vi "Main_Framework.vi"() -> (0 "error out":errorcluster, 3 "output anno":T1(plugin-control))   [LabVIEW 2021, in "Framework_lib.lvlib"]
doc: "This example demonstrates how to call a Python function and pass arguments as numpy arrays. It uses a python function to compute the product of two matrices."
uses:
  QMH/Framework_lib.lvlib
  QMH/QMH_Producer_type.ctl
  FW_Image_resultant_data.ctl
  <vilib>/vision/Image Controls.llb/IMAQ Image.ctl
  QMH/QMH_references_enum.ctl
  FW_Consumer_Data.ctl
  FW_pyAnnotation_parameters.ctl
  FW_producer_Cluster.ctl
  FW_producer_Data.ctl
  FW_Results_Data.ctl
  FW_Frames_Data.ctl
  QMH_producer_enum.ctl
  64de032f-f1bc-4223-962d-436fd60f823b.vi
  a236fdb2-980f-4409-8fc5-f52671132e3e.vi
panel:
  in  "Tab Control":enum32{"Original", "BirdEye", "Final"}(tab)
  out "Input Annotation":T1(plugin-control)
  out "Input SUT":T1(plugin-control)
  out "output SUT":T1(plugin-control)
  out "final 2":T1(plugin-control)
  out "final":T1(plugin-control)
  out "Paused_ann":bool
  out "Paused":bool
  in  "Pause?":bool
  in  "PNG/AVI (F:JPG)":bool
  out "data":T5
  out "Message 2":string
  out "Message":string
  in  "Resume":bool
  out "Waveform Graph":sgl[][](graph)
  in  "Start":bool
  in  "Stop":bool
  out "elapsed_img2arr (ms) 2":u32
  out "elapsed_py (ms) 2":u32
  out "elapsed_py (ms)":u32
  out "elapsed_img2arr (ms)":u32
  in  "name or relative path":path[](array[path])=[path "D:/PELUSO/ITSligo/lectures_MENG/5-Thesis/project/test_hough"]
  out "elapsed_redraw":u32
  # "Main"
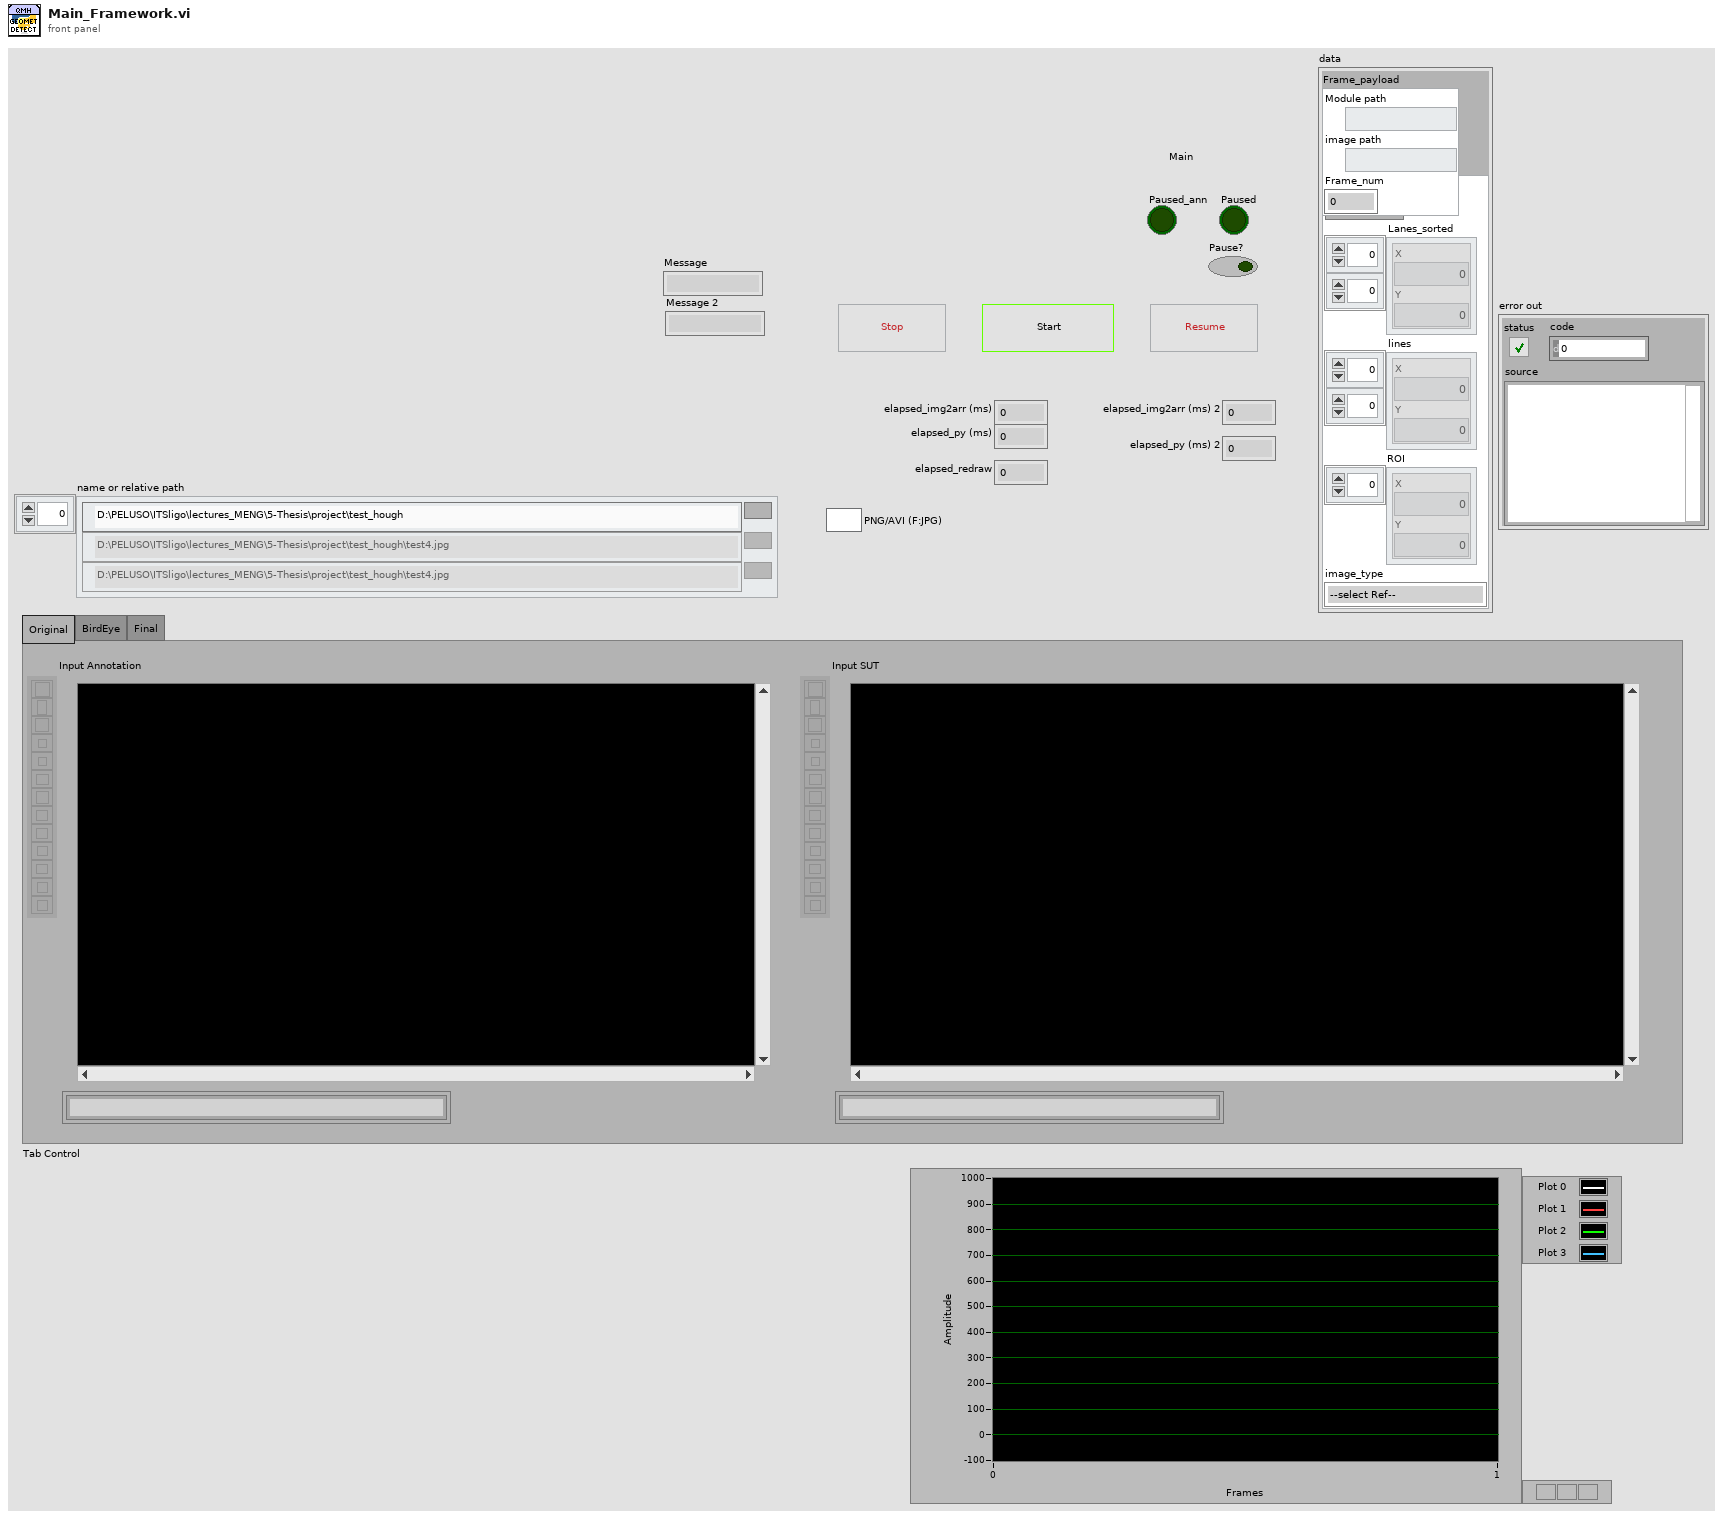
[diagram p1: front panel]
types:
  T1 = typedef "IMAQ Image.ctl" = refnum<image>
  T2 = typedef "Framework_lib.lvlib/QMH_Producer_type.ctl" = cluster{"Module path":path, "image path":path, "Frame_num":u16}
  T3 = typedef "Framework_lib.lvlib/FW_Image_resultant_data.ctl" = cluster{"Image_ref":T1, "Lanes_sorted":cluster{"X":dbl, "Y":dbl}[][], "lines":cluster{"X":dbl, "Y":dbl}[][], "ROI":cluster{"X":dbl, "Y":dbl}[], "image_type":T4}
  T4 = typedef "Framework_lib.lvlib/QMH_references_enum.ctl" = enum16{"--select Ref--", "Consumer_SUT", "Consumer_Annot", "Compute_Results"}
  T5 = cluster{"Frame_payload":T2, "image_resultant":T3}
  T6 = typedef "Framework_lib.lvlib/FW_Consumer_Data.ctl" = cluster{"Py session":refnum<k35>, "Image_orignal":T1, "Image_trans":T1, "ROI_params":T7, "Frame_payload":T2, "image_resultant":T3, "Paused":bool}
  T7 = typedef "Framework_lib.lvlib/FW_pyAnnotation_parameters.ctl" = cluster{"scale_w":dbl, "scale_h":dbl, "offset_X":dbl, "offset_Y":dbl, "Rho":dbl, "Theta":dbl, "Threshold":i32, "min_line_len":i32, "max_line_gap":i32}
  T8 = typedef "Framework_lib.lvlib/FW_Results_Data.ctl" = cluster{"Py session":refnum<k35>, "BirdEyeView_params":cluster{"P1":cluster{"x":i16, "y":i16}, "P2":cluster{"x":i16, "y":i16}, "Alfa":dbl}, "frames_Result":T9[]}
  T9 = typedef "Framework_lib.lvlib/FW_Frames_Data.ctl" = cluster{"Frame_payload":T2, "image_resultant":T3, "Image_Warp_perspective":T1, "Image_Warpped_BW":T1, "Warpped_detected_points":cluster{"X":sgl, "Y":sgl}[][]}
  T10 = cluster{"Global Rectangle":i32[], "Contours":cluster{"Contour Type":u32, "ROI Type":u32, "Points":i32[]}[]}
  T11 = cluster{"scale_w":dbl, "scale_h":dbl, "offset_X":dbl, "offset_Y":dbl, "min_line_len":dbl, "max_line_gap":dbl}
  T12 = typedef "Framework_lib.lvlib/FW_producer_Cluster.ctl" = cluster{"Py session":refnum<k35>, "start_time":u32, "process_running":T13[], "output cluster":T2}
  T13 = typedef "Framework_lib.lvlib/FW_producer_Data.ctl" = cluster{"Queue_Ref":T4, "running":bool}
  T14 = cluster{"Left Lane":cluster{"X":i32, "Y":i32}[], "Right Lane":cluster{"X":i32, "Y":i32}[]}
  T15 = cluster{"Module Path":path, "python_img_array":u8[][][], "Parameters in":variant}
  T16 = typedef "Framework_lib.lvlib/QMH_producer_enum.ctl" = enum16{"Idle", "Initialize", "Shutdown", "ERROR", "Stop", "Start", "Enqueue_frames", "Paused", "Resume"}
  T17 = cluster{"P1":cluster{"x":i16, "y":i16}, "P2":cluster{"x":i16, "y":i16}, "Alfa":dbl}
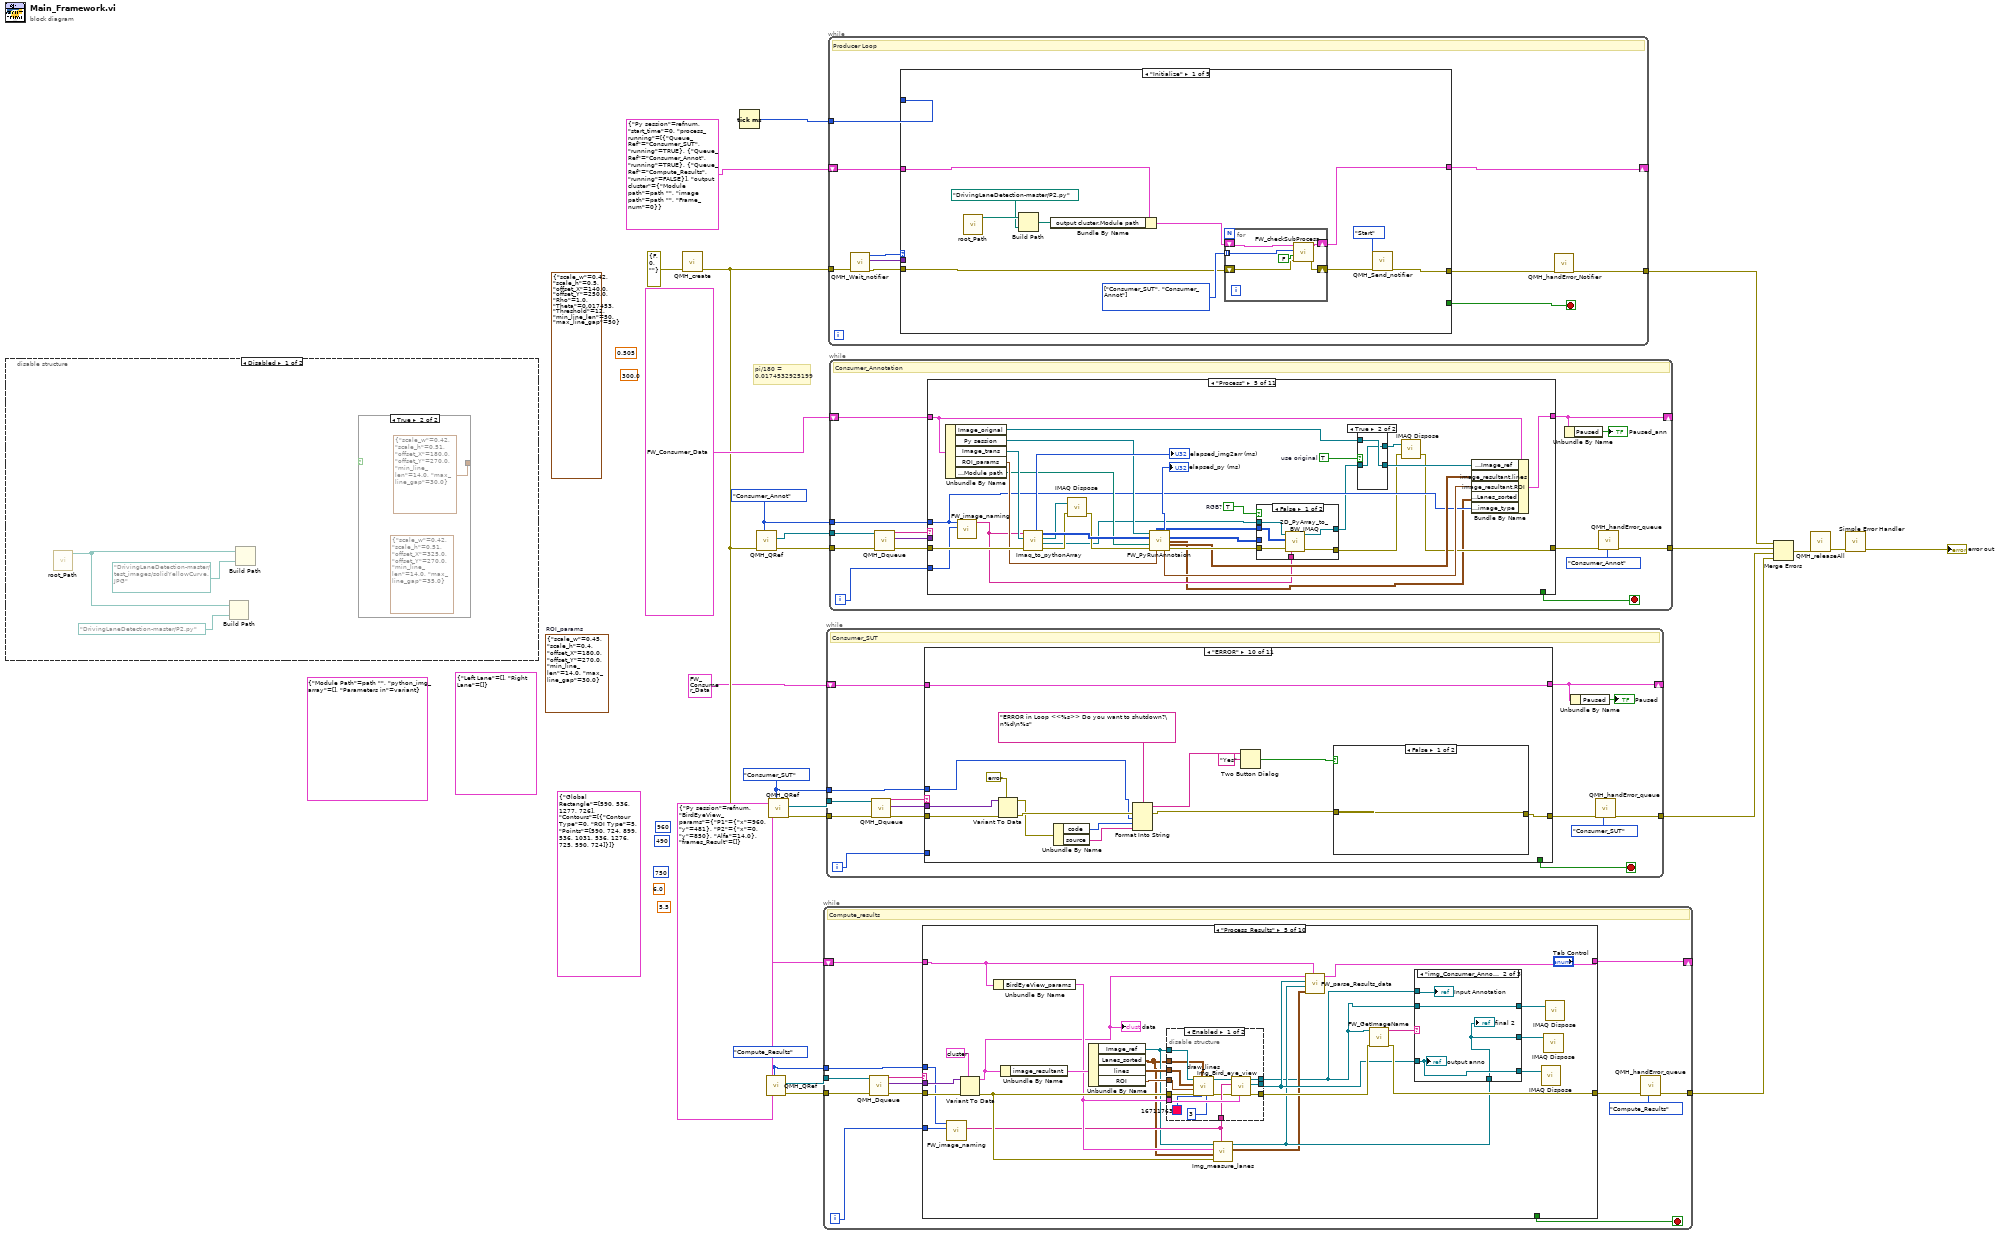
[diagram p0: block diagram]
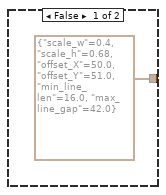
[diagram p2: hidden frame]
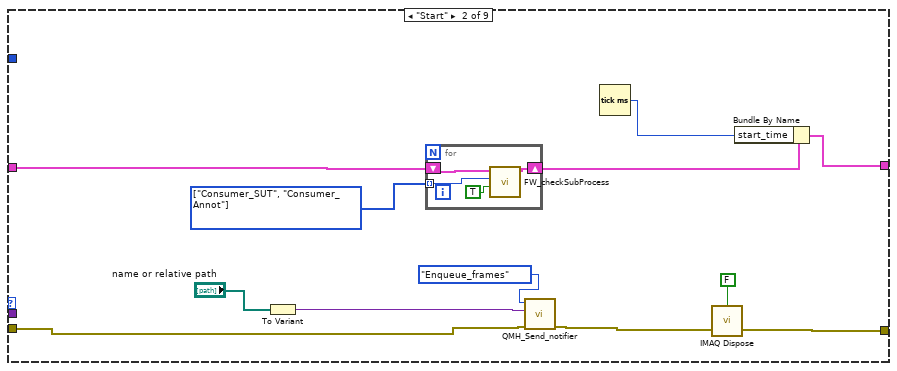
[diagram p4: hidden frame]
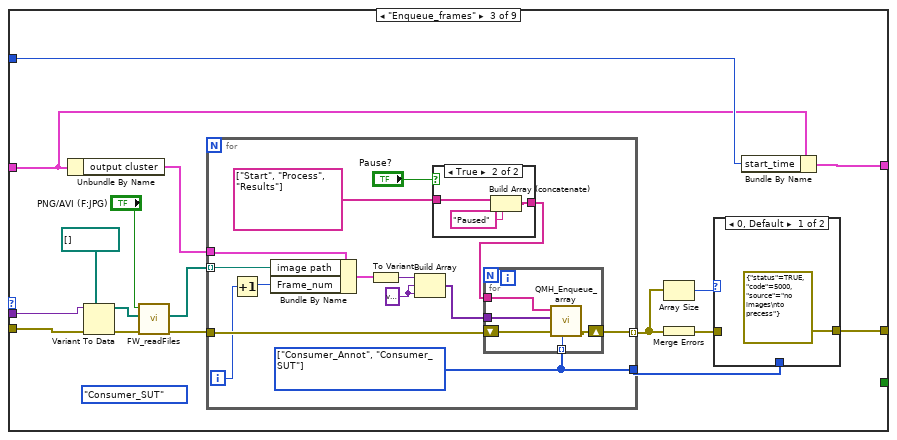
[diagram p5: hidden frame]
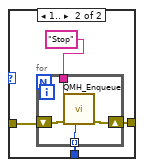
[diagram p6: hidden frame]
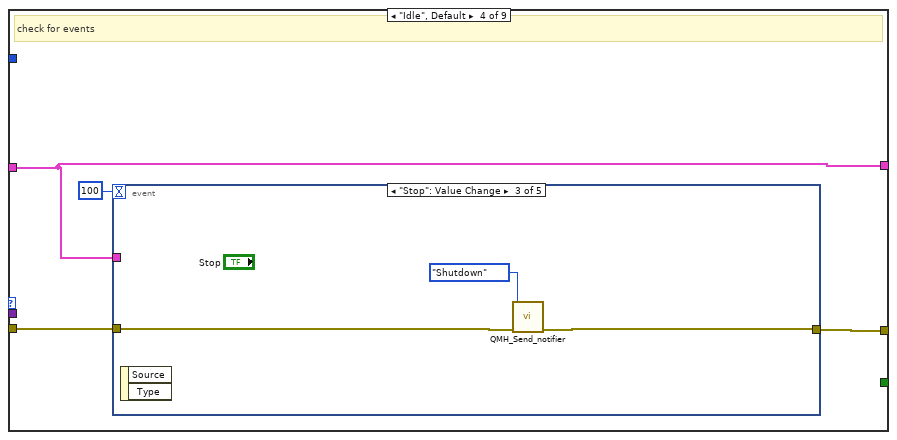
[diagram p8: hidden frame]
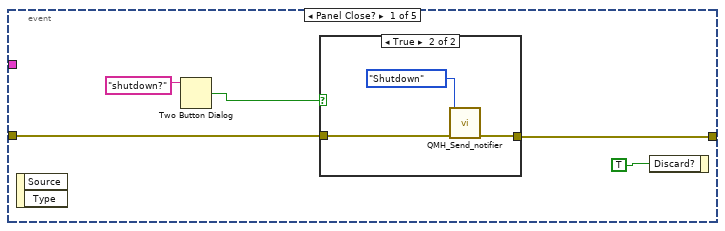
[diagram p9: hidden frame]
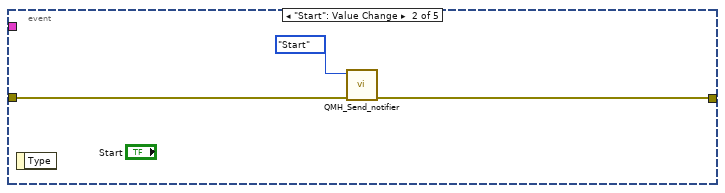
[diagram p11: hidden frame]
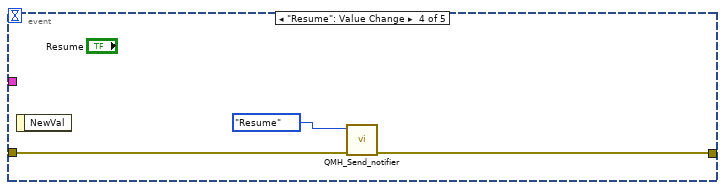
[diagram p12: hidden frame]
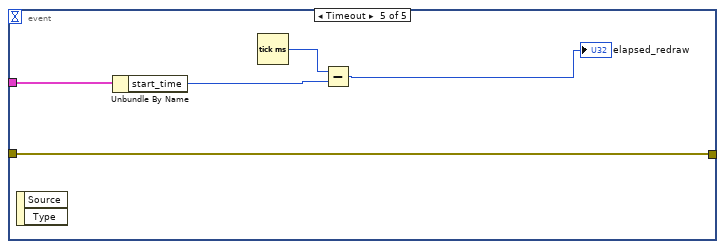
[diagram p13: hidden frame]
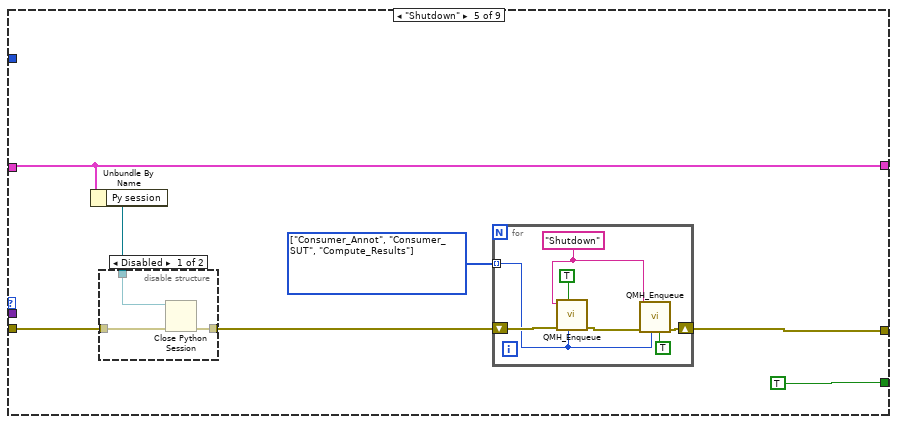
[diagram p14: hidden frame]
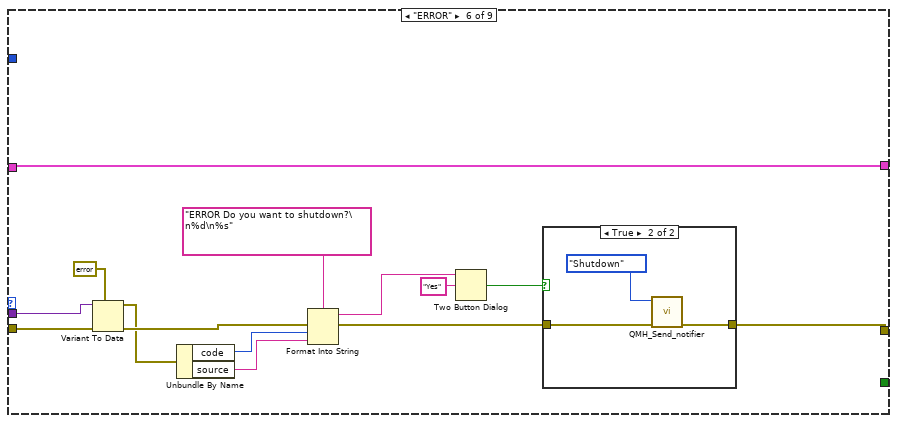
[diagram p16: hidden frame]
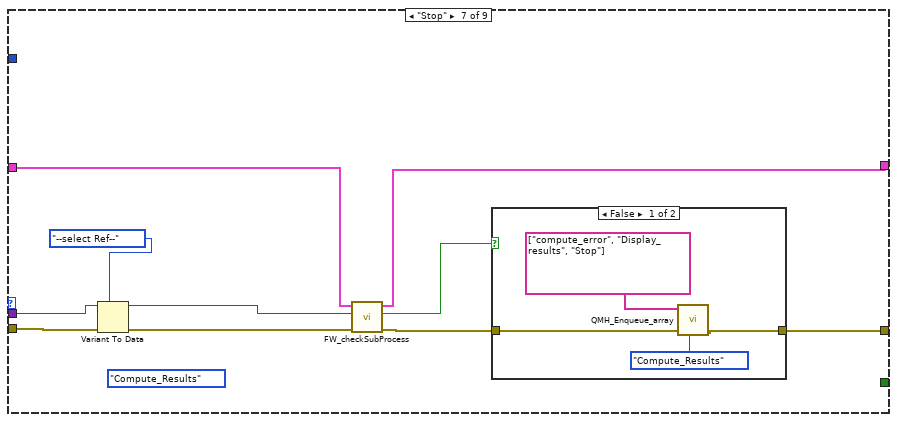
[diagram p18: hidden frame]
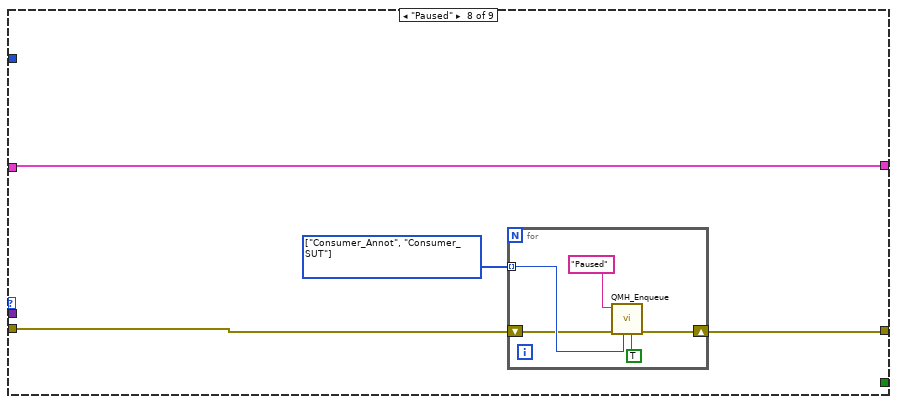
[diagram p20: hidden frame]
diagram:
  (unwired) 0.505 ("scale_h")
  (unwired) 5.5 ("Alfa")
  (unwired) i16 960 ("x")
  (unwired) i16 490 ("y")
  (unwired) 6.0 ("Alfa")
  (unwired) i16 750 ("y")
  (unwired) 300.0 ("offset_Y")
  (unwired) T7 {"scale_w"=0.42, "scale_h"=0.5, "offset_X"=140.0, "offset_Y"=250.0, "Rho"=1.0, "Theta"=0.017453, "Threshold"=12, "min_line_len"=50, "max_line_gap"=50} ("ROI_params")
  w5 = QMH_references_enum."Compute_Results" ("Enum")
  (unwired) T10 {"Global Rectangle"=[590, 536, 1277, 726], "Contours"=[{"Contour Type"=0, "ROI Type"=5, "Points"=[590, 724, 899, 536, 1031, 536, 1276, 725, 590, 724]}]} ("ROI")
  w9 = QMH_references_enum."Consumer_SUT" ("Enum")
  w10 = QMH_references_enum."Consumer_Annot" ("Enum")
  (unwired) T11 {"scale_w"=0.45, "scale_h"=0.4, "offset_X"=180.0, "offset_Y"=270.0, "min_line_len"=14.0, "max_line_gap"=30.0}  # ROI_params
  (unwired) T14 {"Left Lane"=[], "Right Lane"=[]}
  (unwired) T15 {"Module Path"=path "", "python_img_array"=[], "Parameters in"=variant}
  # "pi/180 =\n0.0174532925199"
  n1 = disable-structure shown="Disabled" {
    frame Disabled {
      n2 = call "root_Path.vi"() -> ("name or relative path"=w24:path)  [unwired: 11 in]
      n3 = Build Path(base path=w24, name or relative path=path "DrivingLaneDetection-master/P2.py") -> ()  [unwired: 1 out]
      n4 = Build Path(base path=w24, name or relative path=path "DrivingLaneDetection-master/test_images/solidYellowCurve.JPG") -> ()  [unwired: 1 out]
      n5 = case shown="True" {
        selector: _ -> [_ _]
        tunnel: [T11 {"scale_w"=0.4, "scale_h"=0.68, "offset_X"=50.0, "offset_Y"=51.0, "min_line_len"=16.0, "max_line_gap"=42.0} T11 {"scale_w"=0.42, "scale_h"=0.51, "offset_X"=180.0, "offset_Y"=270.0, "min_line_len"=14.0, "max_line_gap"=30.0}] -> _
        frame False {
        }
        frame True {
          (unwired) T11 {"scale_w"=0.42, "scale_h"=0.51, "offset_X"=325.0, "offset_Y"=270.0, "min_line_len"=14.0, "max_line_gap"=35.0}
        }
      }
    }
    frame Enabled {
    }
  }
  n6 = call "QMH_create.vi"("error in (no error)"=errorcluster {"status"=FALSE, "code"=0, "source"=""}) -> ("error out"=w4:errorcluster)  [unwired: 10 in]
  n7 = Tick Count (ms)() -> (millisecond timer value=w2:u32)
  n8 = call "QMH_QRef.vi"("Enum"=w10, "error in (no error)"=w4) -> ("error out"=w14:errorcluster, "Queue_ref"=w13:refnum<queue>)  [unwired: 7 in, 1 out]
  n9 = call "QMH_QRef.vi"("Enum"=w5, "error in (no error)"=w4) -> ("error out"=w7:errorcluster, "Queue_ref"=w6:refnum<queue>)  [unwired: 7 in, 1 out]
  n10 = call "QMH_QRef.vi"("Enum"=w9, "error in (no error)"=w4) -> ("error out"=w12:errorcluster, "Queue_ref"=w11:refnum<queue>)  [unwired: 7 in, 1 out]
  n11 = while {
    tunnel: w7 -> [w41]
    tunnel: [w33] -> w3
    shift-right: [w36] -> _
    shift-left: T8 {"Py session"=refnum, "BirdEyeView_params"={"P1"={"x"=960, "y"=481}, "P2"={"x"=0, "y"=850}, "Alfa"=14.0}, "frames_Result"=[]} -> [w37]
    tunnel: w6 -> [w31]
    tunnel: w5 -> [w30]
    i -> [w29]
    stop <- w35 stop-if-true
    # "Compute_results"
    n12 = call "QMH_Dqueue.vi"("error in (no error)"=w41, "Queue_ref"=w31) -> ("error out"=w40:errorcluster, "Payload"=w38:variant, "Message"=w39:string)  [unwired: 7 in]
    n13 = case shown="\"Process_Results\"" w39 {
      selector: w39 -> [w42 _ _ _ _ _ _ _ _ _]
      tunnel: w40 -> [w46 w49 w55 w69 w97 w126 w129 w136 w150 w170]
      tunnel: w38 -> [_ _ _ w67 w96 _ _ _ w149 _]
      tunnel: [w45 w49 w53 w70 w88 w126 w129 w135 w152 w169] -> w34
      tunnel: w37 -> [w48 w50 w54 w61 w83 w128 w130 w132 w161 w171]
      tunnel: [w48 w50 w52 w61 w82 w128 w130 w132 w161 w171] -> w36
      tunnel: [_ _ _ _ _ _ _ _ _ TRUE] -> w35
      tunnel: w30 -> [w43 _ _ w62 w91 _ _ w134 w148 _]
      tunnel: w29 -> [_ _ _ w63 w90 _ _ _ _ _]
      frame "", Default {
        n14 = Format Into String(format string="Loop <<%s>> : \nbad message: %s", error in=w46, w43, w42) -> (resulting string=w44:string, error out=w45:errorcluster)  [unwired: 1 in]
        n15 = One Button Dialog(message=w44) -> ()  [unwired: 1 in, 1 out]
      }
      frame "*IDLE*" {
        # "do nothing, just loop through"
      }
      frame "Initialize" {
        n16 = disable-structure shown="Disabled" {
          disable-tunnel: w55 -> [w58 w59]
          disable-tunnel: [w57 w59] -> w53
          disable-tunnel: [w56 _] -> w51
          frame Disabled {
            n17 = call "create python session.vi"("error in (no error)"=w58) -> ("error out"=w57:errorcluster, "session out"=w56:refnum<k35>)  [unwired: 8 in, 1 out]
          }
          frame Enabled {
          }
        }
        n18 = Bundle By Name(cluster=w54, "Py session"=w51) -> (w52:T8)
      }
      frame "Start" {
        w71 = "clear_buffer"  # function name
        n19 = Variant To Data(error in=w69, type=T2 {"Module path"=path "", "image path"=path "", "Frame_num"=0} ("output cluster"), Variant=w67) -> (data=w66:T2, error out=w68:errorcluster)
        n20 = call "FW_image_naming.vi"("Numeric"=w63, "Enum"=w62) -> ()  [unwired: 9 in, 1 out]
        n21 = Unbundle By Name(w61) -> ("Py session"=w60:refnum<k35>)
        n22 = Unbundle By Name(w66) -> ("Module path"=w65:path)  [unwired: 1 out]
        n23 = node(w60, w65, w71, w68) -> (w70:errorcluster)  [unwired: 2 in, 3 out]
      }
      frame "Process_Results" {
        n24 = call "FW_image_naming.vi"("Numeric"=w90, "Enum"=w91) -> ("String"=w84:string)  [unwired: 9 in]
        n25 = Variant To Data(error in=w97, type=T5 {"Frame_payload"={"Module path"=path "", "image path"=path "", "Frame_num"=0}, "image_resultant"={"Image_ref"=refnum, "Lanes_sorted"=[], "lines"=[], "ROI"=[], "image_type"=enum."--select Ref--"}} ("output cluster"), Variant=w96) -> (data=w77:T5, error out=w87:errorcluster)
        "data" <- w77
        n26 = Unbundle By Name(w83) -> ("BirdEyeView_params"=w85:T17)
        n27 = Unbundle By Name(w77) -> ("image_resultant"=w94:T3)
        n28 = Unbundle By Name(w94) -> ("Image_ref"=w81:T1, "Lanes_sorted"=w72:cluster{"X":dbl, "Y":dbl}[][], "lines"=w86:cluster{"X":dbl, "Y":dbl}[][], "ROI"=w93:cluster{"X":dbl, "Y":dbl}[])
        n29 = disable-structure shown="Enabled" {
          disable-tunnel: w93 -> [w111 _]
          disable-tunnel: [w110 w112] -> w89
          disable-tunnel: [w109 w113] -> w73
          disable-tunnel: w87 -> [w108 w112]
          disable-tunnel: w86 -> [w107 _]
          disable-tunnel: w85 -> [w106 _]
          disable-tunnel: w84 -> [w105 _]
          disable-tunnel: w81 -> [w104 w113]
          disable-tunnel: [w103 _] -> w80
          disable-tunnel: w72 -> [w98 _]
          frame Enabled {
            n30 = call "draw_lines.vi"("line_width"=3, "line_Color"=u32 16711763, "Lanes"=w98, "error in (no error)"=w108, "ROI"=w111, "lines"=w107, "Image"=w104) -> ("error out"=w101:errorcluster, "Image out"=w102:T1)  [unwired: 3 in]
            n31 = call "Img_Bird_eye_view.vi"("parameters"=w106, "error in (no error)"=w101, "Image Name"=w105, "img annotation in"=w102) -> ("error out"=w110:errorcluster, "img_corrected"=w103:T1, "img annotation out"=w109:T1)  [unwired: 5 in]
          }
          frame Disabled {
          }
        }
        n32 = call "Img_measure_lanes.vi"("img_name"=w84, "error in (no error)"=w87, "Lanes"=w72, "BirdEyeView_params"=w85, "Image"=w81) -> ("detected_points"=w78:cluster{"X":sgl, "Y":sgl}[][], "Image out"=w79:T1)  [unwired: 4 in, 1 out]
        n33 = call "FW_parse_Results_data.vi"(7:w83, "Warpped_detected_points"=w78, "Image_Warpped_BW"=w79, "Image_Warp_perspective"=w80, "Payload_cluster"=w77) -> ("consumer_loop"=w82:T8)  [unwired: 6 in]
        n34 = call "FW_GetImageName.vi"("error in"=w89, "Image"=w73) -> ("error out"=w88:errorcluster, "before match"=w92:string)  [unwired: 8 in]
        n35 = case shown="\"img_Consumer_Annot\"" w92 {
          tunnel: w80 -> [w116 w121 w122]
          tunnel: w79 -> [w117 w120 w123]
          tunnel: [w116 w121 w123] -> w76
          tunnel: [w117 w120 w122] -> w75
          tunnel: [w115 w119 w124] -> w74
          tunnel: w73 -> [w115 w119 w124]
          tunnel: w73 -> [w114 w118 _]
          frame "img_Consumer_SUT" {
            "output SUT" <- w116
            "final" <- w117
            "Input SUT" <- w114
          }
          frame "img_Consumer_Annot" {
            "output anno" <- w121
            "final 2" <- w120
            "Input Annotation" <- w118
          }
          frame Default {
          }
        }
        n36 = call "IMAQ Dispose"("Image"=w76) -> ()  [unwired: 5 in, 1 out]
        n37 = call "IMAQ Dispose"("Image"=w75) -> ()  [unwired: 5 in, 1 out]
        n38 = call "IMAQ Dispose"("Image"=w74) -> ()  [unwired: 5 in, 1 out]
      }
      frame "compute_error" {
        n39 = Unbundle By Name(w128) -> ("frames_Result"=w127:T9[])
        n40 = call "FW_search_results_array.vi"("frames_Result"=w127) -> ("Waveform Graph"=→"Waveform Graph":sgl[][])  [unwired: 10 in]
      }
      frame "Display_results" {
      }
      frame "Stop" {
        n41 = Unbundle By Name(w132) -> ("Py session"=w131:refnum<k35>)
        n42 = disable-structure shown="Enabled" {
          disable-tunnel: w136 -> [w141 w142]
          disable-tunnel: [w140 w142] -> w133
          disable-tunnel: w131 -> [w139 _]
          frame Disabled {
            n43 = Close Python Session(session in=w139, error in=w141) -> (11:w140:errorcluster)
          }
          frame Enabled {
          }
        }
        n44 = To Variant(anything=w134) -> (Variant=w137:variant)
        n45 = call "QMH_Send_notifier.vi"("error in (no error)"=w133, "Payload"=w137, "Message"=QMH_producer_enum."Shutdown") -> ("error out"=w135:errorcluster)  [unwired: 8 in]
      }
      frame "ERROR" {
        n46 = Variant To Data(error in=w150, type=errorcluster {"status"=FALSE, "code"=0, "source"=""} ("error out"), Variant=w149) -> (data=w157:errorcluster, error out=w160:errorcluster)
        n47 = Unbundle By Name(w157) -> ("code"=w151:i32, "source"=w156:string)
        n48 = Format Into String(format string="ERROR in Loop <<%s>> Do you want to shutdown?\n%d\n%s", error in=w160, w148, w151, w156) -> (resulting string=w155:string, error out=w145:errorcluster)  [unwired: 1 in]
        n49 = Two Button Dialog(message=w155, 2:"Yes" ("T button name (\"OK\")")) -> (T button?=w154:bool)  [unwired: 1 in]
        n50 = call "QMH_Enqueue.vi"("Queue_Ref"=QMH_references_enum."Compute_Results", "Flush (F)"=TRUE, "error in (no error)"=w145, "Message"=".") -> ("error out"=w144:errorcluster)  [unwired: 7 in]
        n51 = case shown="True" w154 {
          tunnel: w144 -> [w162 w166]
          tunnel: [w162 w165] -> w152
          frame False {
          }
          frame True {
            n52 = call "QMH_Enqueue.vi"("Queue_Ref"=QMH_references_enum."Consumer_SUT", "error in (no error)"=w166, "Message"="Shutdown") -> ("error out"=w165:errorcluster)  [unwired: 8 in]
          }
        }
      }
      frame "Shutdown" {
        n53 = call "QMH_Send_notifier.vi"("error in (no error)"=w170, "Message"=QMH_producer_enum."Shutdown") -> ("error out"=w169:errorcluster)  [unwired: 9 in]
      }
    }
    n54 = call "QMH_handError_queue.vi"("Queue_Ref"=QMH_references_enum."Compute_Results", "error in (no error)"=w34) -> ("error out"=w33:errorcluster)  [unwired: 9 in]
  }
  n55 = while {
    tunnel: w12 -> [w185]
    tunnel: [w178] -> w17
    shift-right: [w173] -> _
    shift-left: T6 {"Py session"=refnum, "Image_orignal"=refnum, "Image_trans"=refnum, "ROI_params"={"scale_w"=0.42, "scale_h"=0.45, "offset_X"=140.0, "offset_Y"=300.0, "Rho"=3.0, "Theta"=0.001, "Threshold"=11, "min_line_len"=100, "max_line_gap"=180}, "Frame_payload"={"Module path"=path "", "image path"=path "", "Frame_num"=0}, "image_resultant"={"Image_ref"=refnum, "Lanes_sorted"=[], "lines"=[], "ROI"=[], "image_type"=enum."--select Ref--"}, "Paused"=FALSE} -> [w181]
    tunnel: w11 -> [w176]
    tunnel: w9 -> [w175]
    i -> [w174]
    stop <- w180 stop-if-true
    # "Consumer_SUT"
    n56 = call "QMH_Dqueue.vi"("error in (no error)"=w185, "Queue_ref"=w176) -> ("error out"=w184:errorcluster, "Payload"=w182:variant, "Message"=w183:string)  [unwired: 7 in]
    n57 = case shown="\"ERROR\"" w183 {
      selector: w183 -> [w186 _ _ _ _ _ _ _ _ _ _]
      tunnel: w184 -> [w190 w194 w200 w222 w249 w277 w287 w294 w303 w309 w333]
      tunnel: w182 -> [_ _ _ w220 _ _ _ _ _ w308 _]
      tunnel: [w189 w194 w198 w204 w237 w276 w283 w293 w302 w311 w332] -> w179
      tunnel: w181 -> [w192 w195 w199 w212 w252 w275 w288 w297 w299 w320 w334]
      tunnel: [w192 w195 w197 w217 w243 w275 w280 w290 w299 w320 w334] -> w173
      tunnel: [_ _ _ _ _ _ _ _ _ _ TRUE] -> w180
      tunnel: w175 -> [w187 _ _ w213 w242 _ w281 w291 w301 w307 _]
      tunnel: w174 -> [_ _ _ w214 w245 _ _ _ _ _ _]
      frame "", Default {
        n58 = Format Into String(format string="Loop <<%s>> : \nbad message: %s", error in=w190, w187, w186) -> (resulting string=w188:string, error out=w189:errorcluster)  [unwired: 1 in]
        n59 = One Button Dialog(message=w188) -> ()  [unwired: 1 in, 1 out]
      }
      frame "*IDLE*" {
        # "avoid free spinning"
        # "do nothing, just loop through"
        n60 = Wait (ms)(milliseconds to wait=u32 10) -> ()  [unwired: 1 out]
      }
      frame "Initialize" {
        n61 = call "create python session.vi"("error in (no error)"=w200) -> ("error out"=w198:errorcluster, "session out"=w196:refnum<k35>)  [unwired: 8 in, 1 out]
        n62 = Bundle By Name(cluster=w199, "Py session"=w196) -> (w197:T6)
      }
      frame "Start" {
        w218 = T1 refnum  # ref2
        w224 = "clear_buffer"  # function name
        # "once first function is called\npython loads all libs and objects in memory\nspeedup following calls"
        n63 = Variant To Data(error in=w222, type=T2 {"Module path"=path "", "image path"=path "", "Frame_num"=0} ("output cluster"), Variant=w220) -> (data=w210:T2, error out=w221:errorcluster)
        n64 = call "FW_image_naming.vi"("Numeric"=w214, "Enum"=w213) -> ("String"=w205:string)  [unwired: 9 in]
        n65 = Unbundle By Name(w212) -> ("Py session"=w211:refnum<k35>)
        n66 = Unbundle By Name(w210) -> ("Module path"=w216:path, "image path"=w219:path)
        n67 = node(w211, w216, w224, w221) -> (w223:errorcluster)  [unwired: 2 in, 3 out]
        n68 = call "Open_single_Image.vi"("Image Name"=w205, "error in (no error)"=w223, "appended path"=w219, "Refnum in"=w218) -> ("error out"=w206:errorcluster, "Refnum out"=w202:T1)  [unwired: 6 in]
        n69 = Concatenate Strings(w205, "_trans" ("string")) -> (w207:string)
        n70 = call "Img_PreProcess.vi"("copy_name"=w207, "copy_img"=TRUE, "error in (no error)"=w206, "Original Img"=w202) -> ("error out"=w204:errorcluster, "transformed_out"=w203:T1, "Original Img out"=w201:T1)  [unwired: 5 in]
        n71 = Bundle By Name(cluster=w212, "Frame_payload"=w210, "Image_orignal"=w201, "Image_trans"=w203) -> (w217:T6)
      }
      frame "Process" {
        w236 = TRUE  # RGB?
        w241 = TRUE  # use original
        n72 = Unbundle By Name(w252) -> ("Image_orignal"=w239:T1, "Py session"=w251:refnum<k35>, "Image_trans"=w250:T1, "ROI_params"=w248:T7, "Frame_payload.Module path"=w247:path)
        n73 = call "FW_image_naming.vi"("Numeric"=w245, "Enum"=w242) -> ("String"=w226:string)  [unwired: 9 in]
        n74 = call "Imaq_to_pythonArray.vi"("error in (no error)"=w249, "input(RGB_U32)"=w250, "output ref name"=w226) -> ("error out"=w244:errorcluster, "Image Out"=w232:T1, "image_in"=w246:T1, "python_image"=w254:u8[][][], "elapsed_time"=→"elapsed_img2arr (ms) 2":u32)  [unwired: 4 in]
        n75 = call "IMAQ Dispose"("Image"=w246, "error in (no error)"=w244) -> ("error out"=w225:errorcluster)  [unwired: 4 in]
        n76 = call "FW_PyRunAnnotaion.vi"("Refnum in"=w251, "python_image"=w254, "appended path"=w247, "error in (no error)"=w225, "Parameters in"=w248) -> ("2D_image"=w231:u8[][], "elapsed time"=→"elapsed_py (ms) 2":u32, "Python_img"=w233:u8[][][], "Lanes"=w230:cluster{"X":dbl, "Y":dbl}[][], "lines"=w229:cluster{"X":dbl, "Y":dbl}[][], "trapezoid_ROI"=w228:cluster{"X":dbl, "Y":dbl}[], "error out"=w235:errorcluster)  [unwired: 3 in, 1 out]
        n77 = case shown="False" w236 {
          tunnel: [w260 w266] -> w234
          tunnel: w235 -> [w261 w265]
          tunnel: w233 -> [_ w264]
          tunnel: [w259 w263] -> w227
          tunnel: w232 -> [w258 w262]
          tunnel: w231 -> [w257 _]
          tunnel: w226 -> [w256 _]
          frame False {
            n78 = call "2D_PyArray_to_BW_IMAQ.vi"("Image Name"=w256, "error in (no error)"=w261, "pythonArr_IN"=w257, "Refnum in"=w258) -> ("error out"=w260:errorcluster, "Refnum out"=w259:T1)  [unwired: 5 in, 1 out]
          }
          frame True {
            n79 = call "PyArray_to_IMAQ.vi"("error in (no error)"=w265, "pythonArr_IN"=w264, "Refnum in"=w262) -> ("error out"=w266:errorcluster, "Refnum out"=w263:T1)  [unwired: 6 in, 1 out]
          }
        }
        n80 = case shown="True" w241 {
          tunnel: w227 -> [w268 w269]
          tunnel: w239 -> [w267 w270]
          tunnel: [w268 w270] -> w238
          tunnel: [w267 w269] -> w240
          frame False {
          }
          frame True {
          }
        }
        n81 = call "IMAQ Dispose"("Image"=w240, "error in (no error)"=w234) -> ("error out"=w237:errorcluster)  [unwired: 4 in]
        n82 = Bundle By Name(cluster=w252, "image_resultant.Image_ref"=w238, "image_resultant.lines"=w229, "image_resultant.ROI"=w228, "image_resultant.Lanes_sorted"=w230, "image_resultant.image_type"=w242) -> (w243:T6)
      }
      frame "Results" {
        n83 = Unbundle By Name(w275) -> ("Frame_payload"=w274:T2, "image_resultant"=w273:T3)
        n84 = Bundle("Frame_payload"=w274, "image_resultant"=w273) -> (w272:T5)  [unwired: 1 in]
        n85 = call "QMH_Enqueue.vi"("Queue_Ref"=QMH_references_enum."Compute_Results", "error in (no error)"=w277, "Payload"=w272, "Message"="Process_Results" ("format string")) -> ("error out"=w276:errorcluster)  [unwired: 7 in]
      }
      frame "Paused" {
        # "stall while loop, continue if \"resume\"is sent with high priority"
        n86 = call "QMH_Enqueue.vi"("Priority? (F)"=TRUE, "Queue_Ref"=w281, "error in (no error)"=w287, "Message"="Paused") -> ("error out"=w286:errorcluster)  [unwired: 7 in]
        n87 = call "Stall Data Flow.vim"("value in"=w286, "milliseconds to wait"=u32 500) -> ("value out"=w283:errorcluster)  [unwired: 1 out]
        n88 = Bundle By Name(cluster=w288, "Paused"=TRUE) -> (w280:T6)
      }
      frame "Resume" {
        # "continue processing"
        n89 = call "QMH_QRef.vi"("Enum"=w291, "error in (no error)"=w294) -> ("error out"=w296:errorcluster, "Queue_ref"=w295:refnum<queue>)  [unwired: 7 in, 1 out]
        n90 = call "QMH_Dqueue.vi"("error in (no error)"=w296, "Queue_ref"=w295) -> ("error out"=w293:errorcluster, "Message"=→"Message 2":string)  [unwired: 7 in, 1 out]
        n91 = Bundle By Name(cluster=w297, "Paused"=FALSE) -> (w290:T6)
      }
      frame "Stop" {
        n92 = Unbundle By Name(w299) -> ("Py session"=w298:refnum<k35>)
        n93 = Close Python Session(session in=w298, error in=w303) -> (11:w300:errorcluster)
        n94 = To Variant(anything=w301) -> (Variant=w304:variant)
        n95 = call "QMH_Send_notifier.vi"("error in (no error)"=w300, "Payload"=w304, "Message"=QMH_producer_enum."Stop") -> ("error out"=w302:errorcluster)  [unwired: 8 in]
      }
      frame "ERROR" {
        n96 = Variant To Data(error in=w309, type=errorcluster {"status"=FALSE, "code"=0, "source"=""} ("error out"), Variant=w308) -> (data=w316:errorcluster, error out=w319:errorcluster)
        n97 = Unbundle By Name(w316) -> ("code"=w310:i32, "source"=w315:string)
        n98 = Format Into String(format string="ERROR in Loop <<%s>> Do you want to shutdown?\n%d\n%s", error in=w319, w307, w310, w315) -> (resulting string=w314:string, error out=w306:errorcluster)  [unwired: 1 in]
        n99 = Two Button Dialog(message=w314, 2:"Yes" ("T button name (\"OK\")")) -> (T button?=w313:bool)  [unwired: 1 in]
        n100 = case shown="False" w313 {
          tunnel: [w321 w329] -> w311
          tunnel: w306 -> [w321 w324]
          frame False {
          }
          frame True {
            n101 = call "QMH_Enqueue.vi"("Queue_Ref"=QMH_references_enum."Consumer_SUT", "Flush (F)"=TRUE, "error in (no error)"=w324, "Message"=".") -> ("error out"=w322:errorcluster)  [unwired: 7 in]
            n102 = call "QMH_Enqueue.vi"("Queue_Ref"=QMH_references_enum."Consumer_SUT", "error in (no error)"=w322, "Message"="Shutdown") -> ("error out"=w329:errorcluster)  [unwired: 8 in]
          }
        }
      }
      frame "Shutdown" {
        n103 = call "QMH_Send_notifier.vi"("error in (no error)"=w333, "Message"=QMH_producer_enum."Shutdown") -> ("error out"=w332:errorcluster)  [unwired: 9 in]
      }
    }
    n104 = Unbundle By Name(w173) -> ("Paused"=→"Paused":bool)
    n105 = call "QMH_handError_queue.vi"("Queue_Ref"=QMH_references_enum."Consumer_SUT", "error in (no error)"=w179) -> ("error out"=w178:errorcluster)  [unwired: 9 in]
  }
  n106 = while {
    tunnel: w4 -> [w344]
    tunnel: [w336] -> w19
    shift-right: [w338] -> _
    shift-left: T12 {"Py session"=refnum, "start_time"=0, "process_running"=[{"Queue_Ref"=enum."Consumer_SUT", "running"=TRUE}, {"Queue_Ref"=enum."Consumer_Annot", "running"=TRUE}, {"Queue_Ref"=enum."Compute_Results", "running"=FALSE}], "output cluster"={"Module path"=path "", "image path"=path "", "Frame_num"=0}} -> [w337]
    tunnel: w2 -> [w335]
    stop <- w339 stop-if-true
    # "Producer Loop"
    n107 = call "QMH_Wait_notifier.vi"("error in (no error)"=w344) -> ("error out"=w343:errorcluster, "Payload"=w341:variant, "Message"=w342:T16)  [unwired: 8 in]
    n108 = case shown="\"Initialize\"" w342 {
      tunnel: w343 -> [w347 w366 w391 w429 w460 w485 w498 w506 w515]
      tunnel: w341 -> [_ _ w390 _ _ w483 w497 _ _]
      tunnel: [w346 w363 w386 w428 w458 w480 w499 w507 w516] -> w340
      tunnel: [_ _ _ _ TRUE _ _ _ _] -> w339
      tunnel: [w351 w373 w394 w427 w456 w472 w493 w505 w514] -> w338
      tunnel: w337 -> [w350 w371 w388 w427 w456 w472 w492 w505 w514]
      tunnel: w335 -> [_ _ w393 _ _ _ _ _ _]
      frame "Initialize" {
        w352 = T4[] [enum."Consumer_SUT", enum."Consumer_Annot"] items=["--select Ref--", "Consumer_SUT", "Consumer_Annot", "Compute_Results"] ("Queue_Ref")
        n109 = call "root_Path.vi"() -> ("name or relative path"=w355:path)  [unwired: 11 in]
        n110 = Build Path(base path=w355, name or relative path=path "DrivingLaneDetection-master/P2.py") -> (appended path=w353:path)
        n111 = Bundle By Name(cluster=w350, "output cluster.Module path"=w353) -> (w349:T12)
        n112 = for {
          tunnel: w352 -> [w358] mode=indexing
          shift-right: [w359] -> w351
          shift-left: w349 -> [w361]
          shift-right: [w357] -> w348
          shift-left: w347 -> [w356]
          n113 = call "FW_checkSubProcess.vi"("error in"=w356, "running? (F)"=FALSE, "Sub-process name"=w358, "Cluster"=w361) -> ("error out"=w357:errorcluster, "Cluster out"=w359:T12)  [unwired: 5 in, 1 out]
        }
        n114 = call "QMH_Send_notifier.vi"("error in (no error)"=w348, "Message"=QMH_producer_enum."Start") -> ("error out"=w346:errorcluster)  [unwired: 9 in]
      }
      frame "Start" {
        w370 = T4[] [enum."Consumer_SUT", enum."Consumer_Annot"] items=["--select Ref--", "Consumer_SUT", "Consumer_Annot", "Compute_Results"] ("Queue_Ref")
        n115 = To Variant(anything="name or relative path") -> (Variant=w364:variant)
        n116 = for {
          tunnel: w370 -> [w374] mode=indexing
          shift-right: [w375] -> w372
          shift-left: w371 -> [w377]
          n117 = call "FW_checkSubProcess.vi"("running? (F)"=TRUE, "Sub-process name"=w374, "Cluster"=w377) -> ("Cluster out"=w375:T12)  [unwired: 6 in, 2 out]
        }
        n118 = call "QMH_Send_notifier.vi"("error in (no error)"=w366, "Payload"=w364, "Message"=QMH_producer_enum."Enqueue_frames") -> ("error out"=w369:errorcluster)  [unwired: 8 in]
        n119 = Tick Count (ms)() -> (millisecond timer value=w368:u32)
        n120 = call "IMAQ Dispose"("All Images? (No)"=FALSE, "error in (no error)"=w369) -> ("error out"=w363:errorcluster)  [unwired: 4 in]
        n121 = Bundle By Name(cluster=w372, "start_time"=w368) -> (w373:T12)
      }
      frame "Enqueue_frames" {
        (unwired) QMH_references_enum."Consumer_SUT" ("Enum")
        n122 = Unbundle By Name(w388) -> ("output cluster"=w392:T2)
        n123 = Variant To Data(error in=w391, type=path[] [] ("Path"), Variant=w390) -> (data=w384:path[], error out=w385:errorcluster)
        n124 = call "FW_readFiles.vi"("error in (no error)"=w385, "path(dir/img)"=w384, "JPG/AVI (F:JPG)"="PNG/AVI (F:JPG)") -> ("error out"=w382:errorcluster, "image_path_array_out"=w383:path[])  [unwired: 5 in, 2 out]
        n125 = for {
          tunnel: w392 -> [w417]
          tunnel: [w409] -> w387
          tunnel: w383 -> [w407] mode=indexing
          tunnel: w382 -> [w412]
          tunnel: [w408] -> w380 mode=indexing
          i -> [w411]
          w414 = variant ("element")
          w409 = T4[] [enum."Consumer_Annot", enum."Consumer_SUT"] items=["--select Ref--", "Consumer_SUT", "Consumer_Annot", "Compute_Results"] ("Queue_Ref")
          n126 = Increment(x=w411) -> (x+1=w410:i32)
          n127 = Bundle By Name(cluster=w417, "image path"=w407, "Frame_num"=w410) -> (w416:T2)
          n128 = To Variant(anything=w416) -> (Variant=w415:variant)
          n129 = Build Array(w415, w414, w414) -> (w413:variant[])
          n130 = case shown="True" "Pause?" {
            tunnel: string[] ["Start", "Process", "Results"] ("Message") -> [w418 w421]
            tunnel: [w418 w419] -> w405
            frame False {
            }
            frame True {
              n131 = Build Array (concatenate)(w421, "Paused" ("Message")) -> (w419:string[])
            }
          }
          n132 = for {
            tunnel: w409 -> [w426] mode=indexing
            tunnel: w405 -> [w425]
            tunnel: w413 -> [w424]
            shift-right: [w422] -> w408
            shift-left: w412 -> [w423]
            n133 = call "QMH_Enqueue_array.vi"("Queue_Ref"=w426, "error in (no error)"=w423, "Payload"=w424, "Message"=w425) -> ("error out"=w422:errorcluster)  [unwired: 7 in]
          }
        }
        n134 = Array Size(array=w380) -> (size(s)=w378:i32)
        n135 = Merge Errors(w380) -> (w379:errorcluster)
        n136 = case shown="0, Default" w378 {
          tunnel: w387 -> [_ w399]
          tunnel: [errorcluster {"status"=TRUE, "code"=5000, "source"="no images\nto precess"} ("error IO") w398] -> w386
          tunnel: w379 -> [_ w396]
          frame 0, Default {
          }
          frame 1.. {
            n137 = for {
              tunnel: "Stop" ("Message") -> [w400]
              tunnel: w399 -> [w401] mode=indexing
              shift-right: [w402] -> w398
              shift-left: w396 -> [w403]
              n138 = call "QMH_Enqueue.vi"("Queue_Ref"=w401, "error in (no error)"=w403, "Message"=w400) -> ("error out"=w402:errorcluster)  [unwired: 8 in]
            }
          }
        }
        n139 = Bundle By Name(cluster=w388, "start_time"=w393) -> (w394:T12)
      }
      frame "Idle", Default {
        # "check for events"
        n140 = event shown="[2] \"Stop\": Value Change" {
          selector: _ -> [_ _ _ _ _]
          dyn-events: _ -> [_ _ _ _ _]
          timeout: 100 -> [_ _ _ _ _]
          tunnel: w429 -> [w434 w442 w443 w448 w453]
          tunnel: [w433 w441 w444 w447 w453] -> w428
          tunnel: w427 -> [_ _ _ _ w449]
          event Panel Close? {
            n141 = event-data() -> ()  [unwired: 1 in, 2 out]
            n142 = Two Button Dialog(message="shutdown?") -> (T button?=w431:bool)  [unwired: 2 in]
            n143 = case shown="True" w431 {
              tunnel: w434 -> [w436 w439]
              tunnel: [w436 w438] -> w433
              frame False {
              }
              frame True {
                n144 = call "QMH_Send_notifier.vi"("error in (no error)"=w439, "Message"=QMH_producer_enum."Shutdown") -> ("error out"=w438:errorcluster)  [unwired: 9 in]
              }
            }
            n145 = event-data("Discard?"=TRUE) -> ()  [unwired: 1 in, 1 out]
          }
          event "Start": Value Change {
            n146 = event-data() -> ()  [unwired: 1 in, 1 out]
            n147 = call "QMH_Send_notifier.vi"("error in (no error)"=w442, "Message"=QMH_producer_enum."Start") -> ("error out"=w441:errorcluster)  [unwired: 9 in]
          }
          event "Stop": Value Change {
            n148 = event-data() -> ()  [unwired: 1 in, 2 out]
            n149 = call "QMH_Send_notifier.vi"("error in (no error)"=w443, "Message"=QMH_producer_enum."Shutdown") -> ("error out"=w444:errorcluster)  [unwired: 9 in]
          }
          event "Resume": Value Change {
            n150 = event-data() -> ()  [unwired: 1 in, 1 out]
            n151 = call "QMH_Send_notifier.vi"("error in (no error)"=w448, "Message"=QMH_producer_enum."Resume") -> ("error out"=w447:errorcluster)  [unwired: 9 in]
          }
          event Timeout {
            n152 = event-data() -> ()  [unwired: 1 in, 2 out]
            n153 = Unbundle By Name(w449) -> ("start_time"=w450:u32)
            n154 = Tick Count (ms)() -> (millisecond timer value=w452:u32)
            n155 = Subtract(x=w452, y=w450) -> (x-y=→"elapsed_redraw":u32)
          }
        }
      }
      frame "Shutdown" {
        w454 = T4[] [enum."Consumer_Annot", enum."Consumer_SUT", enum."Compute_Results"] items=["--select Ref--", "Consumer_SUT", "Consumer_Annot", "Compute_Results"] ("Queue_Ref")
        n156 = Unbundle By Name(w456) -> ("Py session"=w455:refnum<k35>)
        n157 = disable-structure shown="Disabled" {
          disable-tunnel: w460 -> [w470 w471]
          disable-tunnel: [w469 w471] -> w457
          disable-tunnel: w455 -> [w468 _]
          frame Disabled {
            n158 = Close Python Session(session in=w468, error in=w470) -> (11:w469:errorcluster)
          }
          frame Enabled {
          }
        }
        n159 = for {
          tunnel: w454 -> [w464] mode=indexing
          shift-right: [w467] -> w458
          shift-left: w457 -> [w466]
          w462 = "Shutdown" ("Message")
          n160 = call "QMH_Enqueue.vi"("Queue_Ref"=w464, "Flush (F)"=TRUE, "error in (no error)"=w466, "Message"=w462) -> ("error out"=w465:errorcluster)  [unwired: 7 in]
          n161 = call "QMH_Enqueue.vi"("Priority? (F)"=TRUE, "Queue_Ref"=w464, "error in (no error)"=w465, "Message"=w462) -> ("error out"=w467:errorcluster)  [unwired: 7 in]
        }
      }
      frame "ERROR" {
        n162 = Variant To Data(error in=w485, type=errorcluster {"status"=FALSE, "code"=0, "source"=""} ("error out"), Variant=w483) -> (data=w478:errorcluster, error out=w484:errorcluster)
        n163 = Unbundle By Name(w478) -> ("code"=w477:i32, "source"=w476:string)
        n164 = Format Into String(format string="ERROR Do you want to shutdown?\n%d\n%s", error in=w484, w477, w476) -> (resulting string=w475:string, error out=w481:errorcluster)  [unwired: 1 in]
        n165 = Two Button Dialog(message=w475, 2:"Yes" ("T button name (\"OK\")")) -> (T button?=w474:bool)  [unwired: 1 in]
        n166 = case shown="True" w474 {
          tunnel: w481 -> [w486 w489]
          tunnel: [w486 w488] -> w480
          frame False {
          }
          frame True {
            n167 = call "QMH_Send_notifier.vi"("error in (no error)"=w489, "Message"=QMH_producer_enum."Shutdown") -> ("error out"=w488:errorcluster)  [unwired: 9 in]
          }
        }
      }
      frame "Stop" {
        (unwired) QMH_references_enum."Compute_Results" ("Enum")
        n168 = Variant To Data(error in=w498, type=QMH_references_enum."--select Ref--" ("Sub-process name"), Variant=w497) -> (data=w490:T4, error out=w495:errorcluster)
        n169 = call "FW_checkSubProcess.vi"("error in"=w495, "Sub-process name"=w490, "Cluster"=w492) -> ("error out"=w494:errorcluster, "any process running"=w496:bool, "Cluster out"=w493:T12)  [unwired: 6 in]
        n170 = case shown="False" w496 {
          tunnel: [w501 w504] -> w499
          tunnel: w494 -> [w502 w504]
          frame False {
            n171 = call "QMH_Enqueue_array.vi"("Queue_Ref"=QMH_references_enum."Compute_Results", "error in (no error)"=w502, "Message"=string[] ["compute_error", "Display_results", "Stop"]) -> ("error out"=w501:errorcluster)  [unwired: 8 in]
          }
          frame True {
          }
        }
      }
      frame "Paused" {
        w508 = T4[] [enum."Consumer_Annot", enum."Consumer_SUT"] items=["--select Ref--", "Consumer_SUT", "Consumer_Annot", "Compute_Results"] ("Queue_Ref")
        n172 = for {
          tunnel: w508 -> [w512] mode=indexing
          shift-right: [w511] -> w507
          shift-left: w506 -> [w510]
          n173 = call "QMH_Enqueue.vi"("Priority? (F)"=TRUE, "Queue_Ref"=w512, "error in (no error)"=w510, "Message"="Paused") -> ("error out"=w511:errorcluster)  [unwired: 7 in]
        }
      }
      frame "Resume" {
        w517 = T4[] [enum."Consumer_Annot", enum."Consumer_SUT"] items=["--select Ref--", "Consumer_SUT", "Consumer_Annot", "Compute_Results"] ("Queue_Ref")
        n174 = for {
          tunnel: w517 -> [w521] mode=indexing
          shift-right: [w520] -> w516
          shift-left: w515 -> [w519]
          n175 = call "QMH_Enqueue.vi"("Priority? (F)"=TRUE, "Queue_Ref"=w521, "error in (no error)"=w519, "Message"="Resume") -> ("error out"=w520:errorcluster)  [unwired: 7 in]
        }
      }
    }
    n176 = call "QMH_handError_Notifier.vi"("error in (no error)"=w340) -> ("error out"=w336:errorcluster)  [unwired: 10 in]
  }
  n177 = while {
    tunnel: w14 -> [w536]
    tunnel: [w529] -> w21
    shift-right: [w524] -> _
    shift-left: T6 {"Py session"=refnum, "Image_orignal"=refnum, "Image_trans"=refnum, "ROI_params"={"scale_w"=0.423, "scale_h"=0.495, "offset_X"=140.0, "offset_Y"=300.0, "Rho"=3.0, "Theta"=0.001, "Threshold"=11, "min_line_len"=100, "max_line_gap"=180}, "Frame_payload"={"Module path"=path "", "image path"=path "", "Frame_num"=0}, "image_resultant"={"Image_ref"=refnum, "Lanes_sorted"=[], "lines"=[], "ROI"=[], "image_type"=enum."--select Ref--"}, "Paused"=FALSE} -> [w532]
    tunnel: w13 -> [w527]
    tunnel: w10 -> [w526]
    i -> [w525]
    stop <- w531 stop-if-true
    # "Consumer_Annotation"
    n178 = call "QMH_Dqueue.vi"("error in (no error)"=w536, "Queue_ref"=w527) -> ("error out"=w535:errorcluster, "Payload"=w533:variant, "Message"=w534:string)  [unwired: 7 in]
    n179 = case shown="\"Process\"" w534 {
      selector: w534 -> [w538 _ _ _ _ _ _ _ _ _ _]
      tunnel: w535 -> [w543 w545 w550 w573 w599 w630 w636 w649 w658 w662 w686]
      tunnel: w533 -> [_ _ _ w571 _ _ _ _ _ w661 _]
      tunnel: [w539 w545 w549 w552 w577 w629 w635 w648 w657 w664 w685] -> w530
      tunnel: w532 -> [w540 w546 w551 w563 w593 w624 w631 w650 w651 w673 w687]
      tunnel: [w540 w546 w548 w568 w592 w624 w632 w643 w651 w673 w687] -> w524
      tunnel: [_ _ _ _ _ _ _ _ _ _ TRUE] -> w531
      tunnel: w526 -> [w537 _ _ w564 w588 _ w634 w645 w654 w660 _]
      tunnel: w525 -> [_ _ _ w565 w595 _ _ _ _ _ _]
      frame "", Default {
        n180 = Format Into String(format string="Loop <<%s>> : \nbad message: %s", error in=w543, w537, w538) -> (resulting string=w541:string, error out=w539:errorcluster)  [unwired: 1 in]
        n181 = One Button Dialog(message=w541) -> ()  [unwired: 1 in, 1 out]
      }
      frame "*IDLE*" {
        # "avoid free spinning"
        # "do nothing, just loop through"
        n182 = Wait (ms)(milliseconds to wait=u32 10) -> ()  [unwired: 1 out]
      }
      frame "Initialize" {
        n183 = call "create python session.vi"("error in (no error)"=w550) -> ("error out"=w549:errorcluster, "session out"=w547:refnum<k35>)  [unwired: 8 in, 1 out]
        n184 = Bundle By Name(cluster=w551, "Py session"=w547) -> (w548:T6)
      }
      frame "Start" {
        w569 = T1 refnum  # ref1
        w575 = "clear_buffer"  # function name
        # "once first function is called\npython loads all libs and objects in memory\nspeedup following calls"
        n185 = Variant To Data(error in=w573, type=T2 {"Module path"=path "", "image path"=path "", "Frame_num"=0} ("output cluster"), Variant=w571) -> (data=w561:T2, error out=w572:errorcluster)
        n186 = call "FW_image_naming.vi"("Numeric"=w565, "Enum"=w564) -> ("String"=w558:string)  [unwired: 9 in]
        n187 = Unbundle By Name(w563) -> ("Py session"=w562:refnum<k35>)
        n188 = Unbundle By Name(w561) -> ("Module path"=w567:path, "image path"=w570:path)
        n189 = node(w562, w567, w575, w572) -> (w574:errorcluster)  [unwired: 2 in, 3 out]
        n190 = call "Open_single_Image.vi"("Image Name"=w558, "error in (no error)"=w574, "appended path"=w570, "Refnum in"=w569) -> ("error out"=w554:errorcluster, "Refnum out"=w560:T1)  [unwired: 6 in]
        n191 = Concatenate Strings(w558, "_trans" ("string")) -> (w556:string)
        n192 = call "Img_PreProcess.vi"("copy_name"=w556, "copy_img"=TRUE, "error in (no error)"=w554, "Original Img"=w560) -> ("error out"=w552:errorcluster, "transformed_out"=w555:T1, "Original Img out"=w553:T1)  [unwired: 5 in]
        n193 = Bundle By Name(cluster=w563, "Frame_payload"=w561, "Image_orignal"=w553, "Image_trans"=w555) -> (w568:T6)
      }
      frame "Process" {
        w580 = TRUE  # use original
        w584 = TRUE  # RGB?
        n194 = Unbundle By Name(w593) -> ("Image_orignal"=w582:T1, "Py session"=w601:refnum<k35>, "Image_trans"=w600:T1, "ROI_params"=w598:T7, "Frame_payload.Module path"=w597:path)
        n195 = call "FW_image_naming.vi"("Numeric"=w595, "Enum"=w588) -> ("String"=w587:string)  [unwired: 9 in]
        n196 = call "Imaq_to_pythonArray.vi"("error in (no error)"=w599, "input(RGB_U32)"=w600, "output ref name"=w587) -> ("error out"=w594:errorcluster, "Image Out"=w586:T1, "image_in"=w596:T1, "python_image"=w604:u8[][][], "elapsed_time"=→"elapsed_img2arr (ms)":u32)  [unwired: 4 in]
        n197 = call "IMAQ Dispose"("Image"=w596, "error in (no error)"=w594) -> ("error out"=w589:errorcluster)  [unwired: 4 in]
        n198 = call "FW_PyRunAnnotaion.vi"("Refnum in"=w601, "python_image"=w604, "appended path"=w597, "error in (no error)"=w589, "Parameters in"=w598) -> ("2D_image"=w585:u8[][], "elapsed time"=→"elapsed_py (ms)":u32, "Python_img"=w602:u8[][][], "Lanes"=w576:cluster{"X":dbl, "Y":dbl}[][], "lines"=w591:cluster{"X":dbl, "Y":dbl}[][], "trapezoid_ROI"=w590:cluster{"X":dbl, "Y":dbl}[], "error out"=w605:errorcluster)  [unwired: 3 in, 1 out]
        n199 = case shown="False" w584 {
          tunnel: [w615 w622] -> w578
          tunnel: w605 -> [w616 w621]
          tunnel: w602 -> [_ w620]
          tunnel: w587 -> [w611 w619]
          tunnel: [w614 w618] -> w583
          tunnel: w586 -> [w613 w617]
          tunnel: w585 -> [w612 _]
          frame False {
            n200 = call "2D_PyArray_to_BW_IMAQ.vi"("Image Name"=w611, "error in (no error)"=w616, "pythonArr_IN"=w612, "Refnum in"=w613) -> ("error out"=w615:errorcluster, "Refnum out"=w614:T1)  [unwired: 5 in, 1 out]
          }
          frame True {
            n201 = call "PyArray_to_IMAQ.vi"("Image Name"=w619, "error in (no error)"=w621, "pythonArr_IN"=w620, "Refnum in"=w617) -> ("error out"=w622:errorcluster, "Refnum out"=w618:T1)  [unwired: 5 in, 1 out]
          }
        }
        n202 = case shown="True" w580 {
          tunnel: w583 -> [w608 w609]
          tunnel: w582 -> [w607 w610]
          tunnel: [w608 w610] -> w581
          tunnel: [w607 w609] -> w579
          frame False {
          }
          frame True {
          }
        }
        n203 = call "IMAQ Dispose"("Image"=w579, "error in (no error)"=w578) -> ("error out"=w577:errorcluster)  [unwired: 4 in]
        n204 = Bundle By Name(cluster=w593, "image_resultant.Image_ref"=w581, "image_resultant.lines"=w591, "image_resultant.ROI"=w590, "image_resultant.Lanes_sorted"=w576, "image_resultant.image_type"=w588) -> (w592:T6)
      }
      frame "Results" {
        n205 = Unbundle By Name(w624) -> ("Frame_payload"=w626:T2, "image_resultant"=w625:T3)
        n206 = Bundle("Frame_payload"=w626, "image_resultant"=w625) -> (w623:T5)  [unwired: 1 in]
        n207 = call "QMH_Enqueue.vi"("Queue_Ref"=QMH_references_enum."Compute_Results", "error in (no error)"=w630, "Payload"=w623, "Message"="Process_Results") -> ("error out"=w629:errorcluster)  [unwired: 7 in]
      }
      frame "Paused" {
        # "stall while loop, continue if \"resume\"is sent with high priority"
        n208 = call "QMH_Enqueue.vi"("Priority? (F)"=TRUE, "Queue_Ref"=w634, "error in (no error)"=w636, "Message"="Paused") -> ("error out"=w640:errorcluster)  [unwired: 7 in]
        n209 = call "Stall Data Flow.vim"("value in"=w640, "milliseconds to wait"=u32 500) -> ("value out"=w635:errorcluster)  [unwired: 1 out]
        n210 = Bundle By Name(cluster=w631, "Paused"=TRUE) -> (w632:T6)
      }
      frame "Resume" {
        # "remove last paused message only"
        n211 = call "QMH_QRef.vi"("Enum"=w645, "error in (no error)"=w649) -> ("error out"=w647:errorcluster, "Queue_ref"=w646:refnum<queue>)  [unwired: 7 in, 1 out]
        n212 = call "QMH_Dqueue.vi"("timeout in ms (-1)"=10, "error in (no error)"=w647, "Queue_ref"=w646) -> ("error out"=w648:errorcluster, "Message"=→"Message":string)  [unwired: 6 in, 1 out]
        n213 = Bundle By Name(cluster=w650, "Paused"=FALSE) -> (w643:T6)
      }
      frame "Stop" {
        n214 = Unbundle By Name(w651) -> ("Py session"=w652:refnum<k35>)
        n215 = Close Python Session(session in=w652, error in=w658) -> (11:w653:errorcluster)
        n216 = To Variant(anything=w654) -> (Variant=w655:variant)
        n217 = call "QMH_Send_notifier.vi"("error in (no error)"=w653, "Payload"=w655, "Message"=QMH_producer_enum."Stop") -> ("error out"=w657:errorcluster)  [unwired: 8 in]
      }
      frame "ERROR" {
        n218 = Variant To Data(error in=w662, type=errorcluster {"status"=FALSE, "code"=0, "source"=""} ("error out"), Variant=w661) -> (data=w669:errorcluster, error out=w672:errorcluster)
        n219 = Unbundle By Name(w669) -> ("code"=w663:i32, "source"=w668:string)
        n220 = Format Into String(format string="ERROR in Loop <<%s>> Do you want to shutdown?\n%d\n%s", error in=w672, w660, w663, w668) -> (resulting string=w667:string, error out=w659:errorcluster)  [unwired: 1 in]
        n221 = Two Button Dialog(message=w667, 2:"Yes" ("T button name (\"OK\")")) -> (T button?=w666:bool)  [unwired: 1 in]
        n222 = case shown="True" w666 {
          tunnel: [w674 w682] -> w664
          tunnel: w659 -> [w674 w677]
          frame False {
          }
          frame True {
            n223 = call "QMH_Enqueue.vi"("Queue_Ref"=QMH_references_enum."Consumer_Annot", "Flush (F)"=TRUE, "error in (no error)"=w677, "Message"=".") -> ("error out"=w675:errorcluster)  [unwired: 7 in]
            n224 = call "QMH_Enqueue.vi"("Queue_Ref"=QMH_references_enum."Consumer_Annot", "error in (no error)"=w675, "Message"="Shutdown") -> ("error out"=w682:errorcluster)  [unwired: 8 in]
          }
        }
      }
      frame "Shutdown" {
        n225 = call "QMH_Send_notifier.vi"("error in (no error)"=w686, "Message"=QMH_producer_enum."Shutdown") -> ("error out"=w685:errorcluster)  [unwired: 9 in]
      }
    }
    n226 = Unbundle By Name(w524) -> ("Paused"=→"Paused_ann":bool)
    n227 = call "QMH_handError_queue.vi"("Queue_Ref"=QMH_references_enum."Consumer_Annot", "error in (no error)"=w530) -> ("error out"=w529:errorcluster)  [unwired: 9 in]
  }
  n228 = Merge Errors(w19, w21, w17, w3) -> (w20:errorcluster)
  n229 = call "QMH_releaseAll.vi"("error in (no error)"=w20) -> ("error out"=w16:errorcluster)  [unwired: 10 in]
  n230 = call <vilib>:"Simple Error Handler.vi"("error in (no error)"=w16) -> ("error out"=→"error out":errorcluster)  [unwired: 4 in, 4 out]
